vi "queue_max_size.vi"() -> ()   [LabVIEW 2021]
panel:
  out "timeout?":bool[](array[boolean])
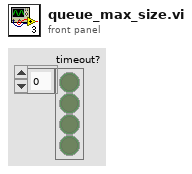
[diagram p1: front panel]
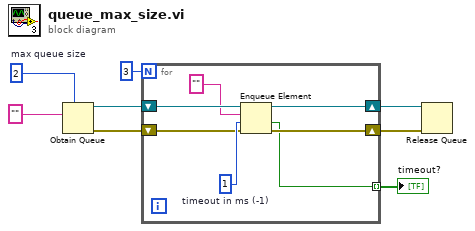
[diagram p0: block diagram]
diagram:
  w8 = 2  # max queue size
  n1 = Obtain Queue(max queue size (-1, unlimited)=w8, element data type="") -> (queue out=w4:refnum<queue>, error out=w2:errorcluster)  [unwired: 3 in, 1 out]
  n2 = for {
    N: 3 -> [_]
    shift-right: [w14] -> w5
    shift-left: w4 -> [w13]
    shift-right: [w15] -> w6
    shift-left: w2 -> [w10]
    tunnel: [w11] -> w3 mode=indexing
    w12 = 1  # timeout in ms (-1)
    n3 = Enqueue Element(queue=w13, element="", timeout in ms (-1)=w12, error in (no error)=w10) -> (queue out=w14:refnum<queue>, timed out?=w11:bool, error out=w15:errorcluster)
  }
  "timeout?" <- w3
  n4 = Release Queue(queue=w5, error in (no error)=w6) -> ()  [unwired: 1 in, 3 out]
